vi "Append Paragraph with Link.vi"(0 "PDF Report":refnum<class "PDF Report Class.lvclass">, 2 "Text":T2={"Text"={"Text"="", "Path"=path "", "Font complete"={"Name"="", "Size"=-1.0, "Color"=0, "Style"={"Bold"=FALSE, "Italic"=FALSE, "Underline"=FALSE, "Strikeout"=FALSE}, "Type"={"Type&direction"=enum."Select", "Embedded"=FALSE, "Encoding"=""}}}, "Link"={"Hyperlink"="", "Font complete"={"Name"="", "Size"=-1.0, "Color"=255, "Style"={"Bold"=FALSE, "Italic"=TRUE, "Underline"=FALSE, "Strikeout"=FALSE}, "Type"={"Type&direction"=enum."Select", "Embedded"=FALSE, "Encoding"=""}}}, "Paragraphe"={" Aligment"=enum."Select", "Line spacing"=enum."Select"}, "Indentation"={"Left"=0.0, "Right"=0.0}}, 11 "error in (no error)":errorcluster, 13 "Image to Add refnum [ ]":T1) -> (4 "PDF Report duplicate":refnum<class "PDF Report Class.lvclass">, 15 "error out":errorcluster)   [LabVIEW 2019, in "Exaprom PDF.lvlib"]
doc: "Appends text with a <B>line feed</B>, at the end, to the PDF report. This text can be <B>aligned</B> (CENTER, JUSTIFY, LEFT, RIGHT) and <B>indented</B>. \n\nIf <B>Font</B> and <B>Pararaph properties</B> are not specified then the <B>Default font</B> and <B>Default paragraph</B> will be use.\n\nThe data type you wire to the <B>Text</B> input determines the polymorphic instance to use.\n\n<B>FRANÇAIS</B>\nAjoute au rapport PDF du texte sous la forme d'un paragraphe terminé avec un \"<B>Line Feed</B>\". Ce texte peut être <B>aligné</B> (CENTER, JUSTIFY, LEFT, RIGHT) et avoir un <B>renfoncement</B> (gauche et droit) pour tout le paragraphe.\n\nSi la police de caractères <B>Font</B> et les propriétés <B>Pararaph properties</B> ne sont pas spécifiés alors la police par défaut <B>Default font</B> et <B>Default paragraph</B> seront utilisées.\n\nLe type de données que vous connectez au terminal <B>Text</B> détermine l'instance polymorphique utilisée.\n\nVersion 2.0\nDeveloped by Jean-Marc Simard\nCopyright © 2013, Exaprom Inc.\nAll rights reserved.\nLicense: BSD\n\nWith iTextSharp 4.1.6 (http://itextsharp.sourceforge.net)\nunder Mozilla Public License Version 1.1\n(http://www.mozilla.org/MPL/MPL-1.1.html)"
uses:
  LV Class/PDF Report Class/PDF Report Class.lvclass
  Controls/Text Controls/Text from String of File and hyperlink.ctl
  Controls/Font Controls/Font complete cluster horizontal.ctl
  Controls/Font Controls/Font size.ctl
  Controls/Font Controls/Font color.ctl
  Controls/Font Controls/Type and encoding.ctl
  Controls/Text Controls/Unicode/Type and run direction.ctl
  Controls/Initialization Controls/Defaut Paragraphe and Line Spacing.ctl
  Controls/Text Controls/Texte alignement.ctl
  Controls/Text Controls/Line spacing.ctl
  Controls/Text Controls/Paragraph indentation.ctl
  Controls/General Controls/Image to Add refnum [ ].ctl
  C:/work/niobrara_lv/labview pdf writer fixing/DLL/itextsharp.dll
  DLL/itextsharp.dll
  Controls/Text Controls/Unicode/Source rub direction.ctl
  Controls/Text Controls/Phrase or paragraph.ctl
  Exaprom PDF.lvlib
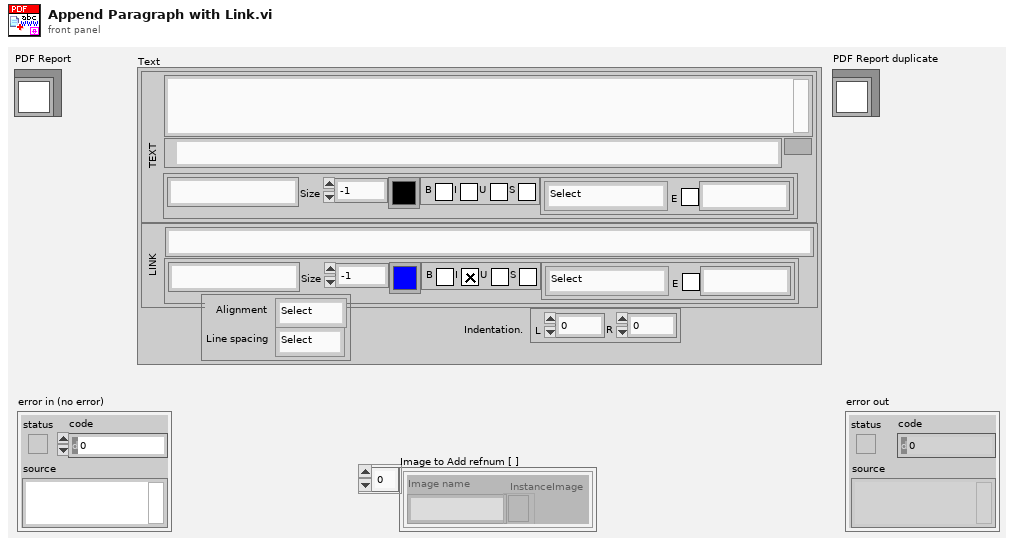
[diagram p1: front panel]
types:
  T1 = typedef "Exaprom PDF.lvlib/Image to Add refnum [ ].ctl" = cluster{"Image name":string, "InstanceImage":refnum<k24>}[]
  T2 = typedef "Exaprom PDF.lvlib/Text from String of File and hyperlink.ctl" = cluster{"Text":cluster{"Text":string, "Path":path, "Font complete":T3}, "Link":cluster{"Hyperlink":string, "Font complete":T3}, "Paragraphe":T8, "Indentation":T11}
  T3 = typedef "Exaprom PDF.lvlib/Font complete cluster horizontal.ctl" = cluster{"Name":string, "Size":T4, "Color":T5, "Style":cluster{"Bold":bool, "Italic":bool, "Underline":bool, "Strikeout":bool}, "Type":T6}
  T4 = typedef "Exaprom PDF.lvlib/Font size.ctl" = sgl
  T5 = typedef "Exaprom PDF.lvlib/Font color.ctl" = u32
  T6 = typedef "Exaprom PDF.lvlib/Type and encoding.ctl" = cluster{"Type&direction":T7, "Embedded":bool, "Encoding":string}
  T7 = typedef "Exaprom PDF.lvlib/Type and run direction.ctl" = enum16{"Select", "ASCII", "UTF-16", "UTF-16 (default)", "UTF-16 (LTR)", "UTF-16 (RTL)"}
  T8 = typedef "Exaprom PDF.lvlib/Defaut Paragraphe and Line Spacing.ctl" = cluster{" Aligment":T9, "Line spacing":T10}
  T9 = typedef "Exaprom PDF.lvlib/Texte alignement.ctl" = enum16{"Select", "CENTER", "JUSTIFY", "LEFT", "RIGHT"}
  T10 = typedef "Exaprom PDF.lvlib/Line spacing.ctl" = enum16{"Select", "1.0", "1.5", "2.0"}
  T11 = typedef "Exaprom PDF.lvlib/Paragraph indentation.ctl" = cluster{"Left":sgl, "Right":sgl}
  T12 = typedef "Exaprom PDF.lvlib/Source rub direction.ctl" = enum16{"Chapter", "Paragraph", "Phrase", "pdfpcell"}
  T13 = typedef "Exaprom PDF.lvlib/Phrase or paragraph.ctl" = enum16{"Add to Phrase", "Add to Paragraph", "Create Phrase", "Create Paragraph"}
  T14 = typedef "Exaprom PDF.lvlib/Text type.ctl" = enum16{"empty", "Text", "Hyperlink"}
  T15 = cluster{"Text type":T14, "Text":string, "Hyperlink":string}[]
  T16 = typedef "Exaprom PDF.lvlib/Page dimensions.ctl" = cluster{"Start at page":i32, "Page Size":T17, "Orientation":T18, "widht":sgl, "height":sgl, "Margin left":sgl, "Margin right":sgl, "Margin top":sgl, "Margin bottom":sgl, "X0":sgl, "X1":sgl, "Y0":sgl, "Y1":sgl}
  T17 = typedef "Exaprom PDF.lvlib/Page size.ctl" = i32
  T18 = typedef "Exaprom PDF.lvlib/Page Orientation.ctl" = enum16{"Portrait", "Landscape"}
  T19 = typedef "Exaprom PDF.lvlib/Unit.ctl" = enum16{"inch", "mm"}
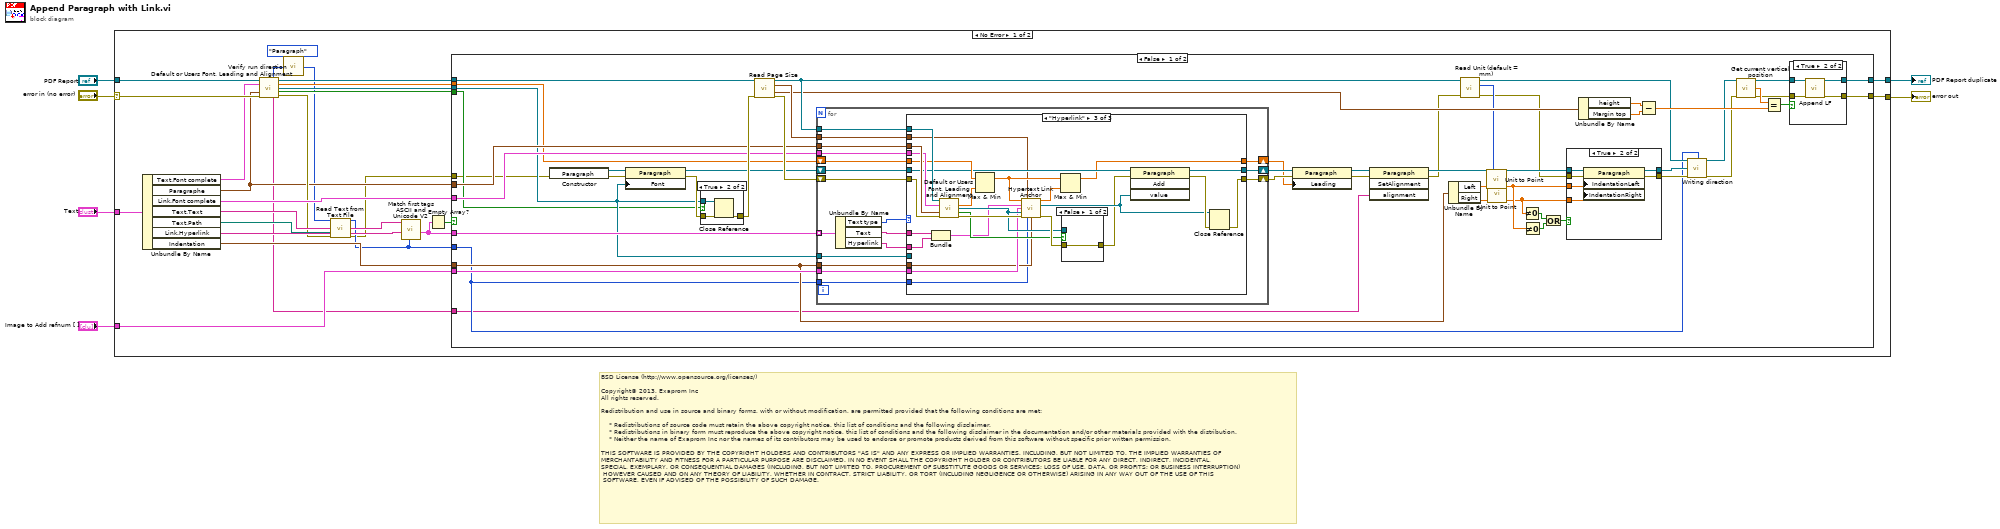
[diagram p0: block diagram]
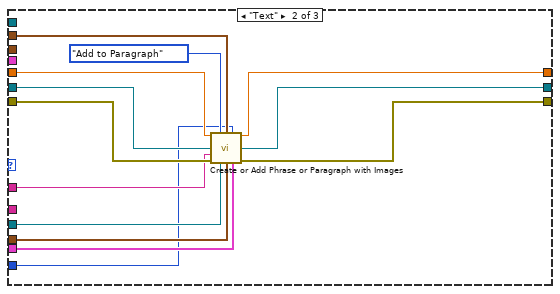
[diagram p4: hidden frame]
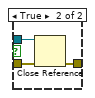
[diagram p5: hidden frame]
diagram:
  # "BSD License (http://www.opensource.org/licenses/)\n\nCopyright© 2013, Exaprom Inc\nAll rights reserved.\n\nRedistribution and use in source and binary forms, with or without modification, are permitted provided that the following conditions are met:\n\n    * Redistributions of source code must retain the above copyright notice, this list of conditions and the following disclaimer.\n    * Redistributions in binary form must reproduce the above copyright notice, this list of conditions and the following disclaimer in the documentation and/or other materials provided with the distribution.\n    * Neither the name of Exaprom Inc nor the names of its contributors may be used to endorse or promote products derived from this software without specific prior written permission.\n\nTHIS SOFTWARE IS PROVIDED BY THE COPYRIGHT HOLDERS AND CONTRIBUTORS \"AS IS\" AND ANY EXPRESS OR IMPLIED WARRANTIES, INCLUDING, BUT NOT LIMITED TO, THE IMPLIED WARRANTIES OF \nMERCHANTABILITY AND FITNESS FOR A PARTICULAR PURPOSE ARE DISCLAIMED. IN NO EVENT SHALL THE COPYRIGHT HOLDER OR CONTRIBUTORS BE LIABLE FOR ANY DIRECT, INDIRECT, INCIDENTAL,\nSPECIAL, EXEMPLARY, OR CONSEQUENTIAL DAMAGES (INCLUDING, BUT NOT LIMITED TO, PROCUREMENT OF SUBSTITUTE GOODS OR SERVICES; LOSS OF USE, DATA, OR PROFITS; OR BUSINESS INTERRUPTION)\n HOWEVER CAUSED AND ON ANY THEORY OF LIABILITY, WHETHER IN CONTRACT, STRICT LIABILITY, OR TORT (INCLUDING NEGLIGENCE OR OTHERWISE) ARISING IN ANY WAY OUT OF THE USE OF THIS\n SOFTWARE, EVEN IF ADVISED OF THE POSSIBILITY OF SUCH DAMAGE."
  n1 = case shown="No Error" "error in (no error)" {
    selector: "error in (no error)" -> [w20 w170]
    tunnel: [w30 w170] -> w6
    tunnel: "PDF Report" -> [w19 w169]
    tunnel: [w31 w169] -> w3
    tunnel: "Text" -> [w33 _]
    tunnel: "Image to Add refnum [ ]" -> [w28 _]
    frame No Error {
      n2 = Unbundle By Name(w33) -> ("Text.Font complete"=w16:T3, "Paragraphe"=w15:T8, "Link.Font complete"=w25:T3, "Text.Text"=w22:string, "Text.Path"=w24:path, "Link.Hyperlink"=w29:string, "Indentation"=w32:T11)
      n3 = call "Default or Users Font, Leading and Alignment.vi"("PDF Report"=w19, "Font"=w16, "Paragraphe cluster"=w15, "error in (no error)"=w20) -> ("Type and run direction"=w14:T7, "PDF Report duplicate"=w17:refnum<class "PDF Report Class.lvclass">, "Leading"=w13:T4, "Font Ref"=w12:refnum<k24>, "Close Font Ref"=w11:bool, "Aligment"=w10:string, "error out"=w18:errorcluster)  [unwired: 5 out]
      n4 = call "Verify run direction.vi"("Source"=Source_rub_direction."Paragraph", "Type&direction IN"=w14) -> ("Type&direction OUT"=w8:T7)  [unwired: 2 in]
      n5 = call "Read Text from Text File.vi"("Text and direction IN"=w8, "Text IN"=w22, "Path"=w24, "error in (no error)"=w18) -> ("Text and direction OUT"=w21:T7, "Text OUT"=w23:string, "error out"=w9:errorcluster)  [unwired: 9 in]
      n6 = call "Match first tags ASCII and Unicode V2.vi"("Type and run direction"=w21, "Hyperlink"=w29, "Text"=w23) -> ("Array"=w26:T15)  [unwired: 2 in, 6 out]
      n7 = Empty Array?(array=w26) -> (empty?=w27:bool)
      n8 = case shown="False" w27 {
        tunnel: w32 -> [w54 _]
        tunnel: [w67 w168] -> w31
        tunnel: [w65 w167] -> w30
        tunnel: w17 -> [w34 w168]
        tunnel: w26 -> [w58 _]
        tunnel: w28 -> [w56 _]
        tunnel: w15 -> [w55 _]
        tunnel: w25 -> [w51 _]
        tunnel: w21 -> [w40 _]
        tunnel: w13 -> [w39 _]
        tunnel: w12 -> [w38 _]
        tunnel: w11 -> [w37 _]
        tunnel: w10 -> [w36 _]
        tunnel: w9 -> [w35 w167]
        frame False {
          n9 = constructor class="Paragraph"(error in=w35) -> (reference out=w62:refnum<k24>, error out=w61:errorcluster)  [unwired: 2 in, 1 out]
          n10 = property class="Paragraph"(reference=w62, error in=w61, "Font"=w38) -> (reference out=w60:refnum<k24>, error out=w49:errorcluster)
          n11 = case shown="True" w37 {
            tunnel: [w85 w88] -> w82
            tunnel: w49 -> [w85 w87]
            tunnel: w38 -> [_ w86]
            frame False {
            }
            frame True {
              n12 = Close Reference(reference=w86, error in (no error)=w87) -> (error out=w88:errorcluster)
            }
          }
          n13 = call "Read Page Size.vi"("PDF Report"=w34, "error in (no error)"=w82) -> ("PDF Report duplicate"=w53:refnum<class "PDF Report Class.lvclass">, "Text zone (points)"=w52:cluster{"widht":sgl, "height":sgl}, "Page (points)"=w50:T16, "error out"=w83:errorcluster)  [unwired: 10 out]
          n14 = for {
            tunnel: w58 -> [w106] mode=indexing
            shift-right: [w99] -> w84
            shift-left: w83 -> [w105]
            shift-right: [w102] -> w59
            shift-left: w60 -> [w103]
            shift-right: [w97] -> w57
            shift-left: w39 -> [w98]
            tunnel: w56 -> [w96]
            tunnel: w51 -> [w95]
            tunnel: w55 -> [w94]
            tunnel: w53 -> [w93]
            tunnel: w52 -> [w92]
            tunnel: w54 -> [w91]
            tunnel: w38 -> [w90]
            tunnel: w40 -> [w89]
            n15 = Unbundle By Name(w106) -> ("Text type"=w104:T14, "Text"=w101:string, "Hyperlink"=w100:string)
            n16 = case shown="\"Hyperlink\"" w104 {
              tunnel: [w109 w120 w135] -> w102
              tunnel: w94 -> [_ _ w141]
              tunnel: w95 -> [_ _ w140]
              tunnel: w93 -> [_ _ w139]
              tunnel: w105 -> [w108 w122 w132]
              tunnel: w103 -> [w109 w119 w133]
              tunnel: [w108 w121 w134] -> w99
              tunnel: w96 -> [_ w112 w136]
              tunnel: w98 -> [w107 w116 w138]
              tunnel: [w107 w115 w126] -> w97
              tunnel: w101 -> [_ w117 w131]
              tunnel: w100 -> [_ _ w130]
              tunnel: w92 -> [_ w114 w125]
              tunnel: w91 -> [_ w113 w124]
              tunnel: w90 -> [_ w111 _]
              tunnel: w89 -> [_ w110 w123]
              frame "empty", Default {
              }
              frame "Text" {
                n17 = call "Create or Add Phrase or Paragraph with Images.vi"("Leading"=w116, "Phrase or paragraph"=Phrase_or_paragraph."Add to Paragraph", "Text zone (points)"=w114, "Character type"=w110, "Paragraph refnum IN"=w119, "Text"=w117, "error in (no error)"=w122, "Font refnum"=w111, "Paragraph indentation (points)"=w113, "Image to Add refnum [ ]"=w112) -> ("Leading duplicate"=w115:sgl, "Paragraph refnum OUT"=w120:refnum<k24>, "error out"=w121:errorcluster)  [unwired: 1 in, 2 out]
              }
              frame "Hyperlink" {
                n18 = Bundle("Text"=w131, "Hyperlink"=w130) -> (w129:cluster{"Text":string, "Hyperlink":string})  [unwired: 1 out]
                n19 = call "Default or Users Font, Leading and Alignment.vi"("PDF Report"=w139, "Font"=w140, "Paragraphe cluster"=w141, "error in (no error)"=w132) -> ("Leading"=w137:T4, "Font Ref"=w143:refnum<k24>, "Close Font Ref"=w142:bool, "error out"=w146:errorcluster)  [unwired: 8 out]
                n20 = Max & Min(x=w138, y=w137) -> (max(x,y)=w128:T4)  [unwired: 1 out]
                n21 = call "Hypertext Link Anchor.vi"("Leading"=w128, "Text zone (points)"=w125, "Hyperlink"=w129, "Image to Add refnum [ ]"=w136, "Font refnum"=w143, "error in (no error)"=w146, "Type and run direction"=w123, "Paragraph indentation (points)"=w124) -> ("Leading OUT"=w127:sgl, "Anchor"=w147:refnum<k24>, "error out"=w145:errorcluster)  [unwired: 1 in, 4 out]
                n22 = Max & Min(x=w128, y=w127) -> (max(x,y)=w126:T4)  [unwired: 1 out]
                n23 = case shown="False" w142 {
                  tunnel: [w149 w152] -> w144
                  tunnel: w145 -> [w149 w151]
                  tunnel: w143 -> [_ w150]
                  frame False {
                  }
                  frame True {
                    n24 = Close Reference(reference=w150, error in (no error)=w151) -> (error out=w152:errorcluster)
                  }
                }
                n25 = invoke class="Paragraph" method="Add"(reference=w133, error in=w144, "value"=w147) -> (reference out=w135:refnum<k24>, error out=w148:errorcluster)  [unwired: 1 in, 2 out]
                n26 = Close Reference(reference=w147, error in (no error)=w148) -> (error out=w134:errorcluster)
              }
            }
          }
          n27 = property class="Paragraph"(reference=w59, error in=w84, "Leading"=w57) -> (reference out=w63:refnum<k24>, error out=w73:errorcluster)
          n28 = invoke class="Paragraph" method="SetAlignment"(reference=w63, error in=w73, "alignment"=w36) -> (reference out=w76:refnum<k24>, error out=w47:errorcluster)  [unwired: 1 in, 2 out]
          n29 = Unbundle By Name(w54) -> ("Left"=w80:sgl, "Right"=w81:sgl)
          n30 = call-dynamic "Read Unit (default = mm).vi"("error in (no error)"=w47, "PDF Report Class in"=w53) -> ("error out"=w43:errorcluster, "Unit (default = mm)"=w48:T19, "PDF Report Class out"=w42:refnum<class "PDF Report Class.lvclass">)  [unwired: 7 in]
          n31 = call "Unit to Point.vi"("X unit"=w80, "Unit (default = mm)"=w48) -> ("X point"=w75:sgl)  [unwired: 7 out]
          n32 = call "Unit to Point.vi"("X unit"=w81, "Unit (default = mm)"=w48) -> ("X point"=w74:sgl)  [unwired: 7 out]
          n33 = Not Equal To 0?(x=w74) -> (x != 0?=w78:bool)
          n34 = Not Equal To 0?(x=w75) -> (x != 0?=w77:bool)
          n35 = Or(x=w78, y=w77) -> (x .or. y?=w79:bool)
          n36 = case shown="True" w79 {
            tunnel: w76 -> [w160 w166]
            tunnel: w43 -> [w159 w165]
            tunnel: [w159 w164] -> w46
            tunnel: [w160 w163] -> w41
            tunnel: w75 -> [_ w162]
            tunnel: w74 -> [_ w161]
            frame False {
            }
            frame True {
              n37 = property class="Paragraph"(reference=w166, error in=w165, "IndentationLeft"=w162, "IndentationRight"=w161) -> (reference out=w163:refnum<k24>, error out=w164:errorcluster)
            }
          }
          n38 = Unbundle By Name(w50) -> ("height"=w71:sgl, "Margin top"=w70:sgl)
          n39 = Subtract(x=w71, y=w70) -> (x-y=w68:sgl)
          n40 = call "Writing direction.vi"("PDF Report IN"=w42, "Text type"=w40, "Paragraph refnum"=w41, "error in (no error)"=w46) -> ("PDF Report OUT"=w44:refnum<class "PDF Report Class.lvclass">, "error out"=w45:errorcluster)  [unwired: 10 in]
          n41 = call "Get current vertical position.vi"("PDF Report In"=w44, "error in (no error)"=w45) -> ("PDF Report duplicate"=w72:refnum<class "PDF Report Class.lvclass">, "GetVerticalPosition (points)"=w69:sgl, "error out"=w66:errorcluster)  [unwired: 1 in, 10 out]
          n42 = Equal?(x=w69, y=w68) -> (x = y?=w64:bool)
          n43 = case shown="True" w64 {
            tunnel: w72 -> [w154 w158]
            tunnel: [w154 w157] -> w67
            tunnel: w66 -> [w153 w156]
            tunnel: [w153 w155] -> w65
            frame False {
            }
            frame True {
              n44 = call "Append LF.vi"("PDF Report IN"=w158, "error in (no error)"=w156) -> ("PDF Report duplicate"=w157:refnum<class "PDF Report Class.lvclass">, "error out"=w155:errorcluster)  [unwired: 2 in, 10 out]
            }
          }
        }
        frame True {
        }
      }
    }
    frame Error {
    }
  }
  "error out" <- w6
  "PDF Report duplicate" <- w3
